vi "Create Unique SheetID.vi"(8 "error in":errorcluster, 11 "Sheets in":refnum<k24>) -> (0 "error out":errorcluster, 2 "Unique SheetID":u32, 3 "Sheets out":refnum<k24>)   [LabVIEW 2019, in "Open Xml.lvlib"]
uses:
  Open Xml.lvlib
  D:/git/Open-Xml-LabVIEW/Source/DocumentFormat.OpenXml.dll
  DocumentFormat.OpenXml.dll
  D:/git/Open-Xml-LabVIEW/Source/DocumentFormat.OpenXml.Framework.dll
  DocumentFormat.OpenXml.Framework.dll
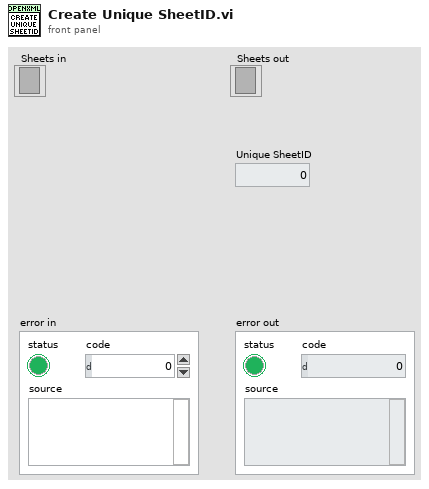
[diagram p1: front panel]
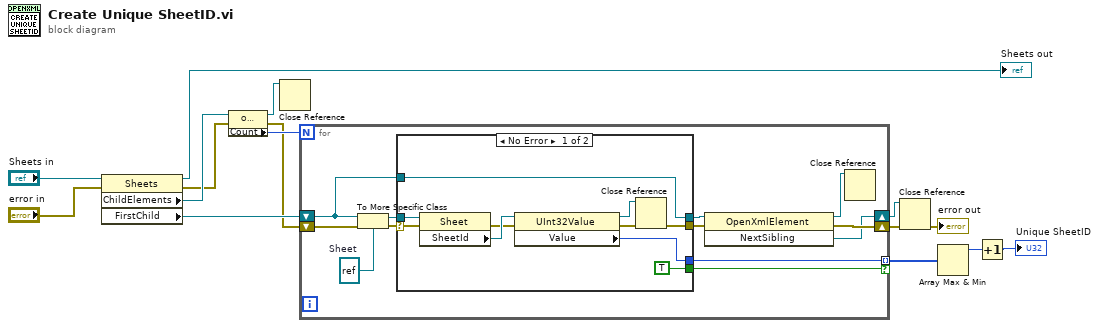
[diagram p0: block diagram]
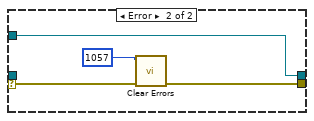
[diagram p2: hidden frame]
diagram:
  n1 = property class="Sheets"(reference="Sheets in", error in="error in") -> (reference out=→"Sheets out":refnum<k24>, error out=w9:errorcluster, "ChildElements"=w14:refnum<k24>, "FirstChild"=w11:refnum<k24>)
  n2 = property class="OpenXmlElementList"(reference=w14, error in=w9) -> (reference out=w4:refnum<k24>, error out=w10:errorcluster, "Count"=w12:i32)
  n3 = Close Reference(reference=w4) -> ()  [unwired: 1 in, 1 out]
  n4 = for {
    N: w12 -> [_]
    tunnel: [w24] -> w8 mode=indexing if=w23
    shift-right: [w20] -> w5
    shift-left: w10 -> [w19]
    shift-right: [w16] -> w1
    shift-left: w11 -> [w18]
    w27 = refnum<k24> refnum  # Sheet
    n5 = To More Specific Class(target class=w27, reference=w18, error in=w19) -> (specific class reference=w25:refnum<k24>, error out=w26:errorcluster)
    n6 = case shown="No Error" w26 {
      selector: w26 -> [w34 w41]
      tunnel: w25 -> [w37 _]
      tunnel: [w28 _] -> w24
      tunnel: [TRUE _] -> w23
      tunnel: [w30 w40] -> w22
      tunnel: [w33 w38] -> w21
      tunnel: w18 -> [w33 w38]
      frame No Error {
        n7 = property class="Sheet"(reference=w37, error in=w34) -> (error out=w32:errorcluster, "SheetId"=w36:refnum<k24>)  [unwired: 1 out]
        n8 = property class="UInt32Value"(reference=w36, error in=w32) -> (reference out=w29:refnum<k24>, error out=w31:errorcluster, "Value"=w28:u32)
        n9 = Close Reference(reference=w29, error in (no error)=w31) -> (error out=w30:errorcluster)
      }
      frame Error {
        n10 = call <vilib>:"Clear Errors.vi"("error in (no error)"=w41, "specific error code to clear (0: all)"=1057) -> ("error out"=w40:errorcluster)  [unwired: 4 in, 1 out]
      }
    }
    n11 = invoke class="OpenXmlElement" method="NextSibling"(reference=w21, error in=w22) -> (reference out=w17:refnum<k24>, error out=w20:errorcluster, "NextSibling"=w16:refnum<k24>)  [unwired: 1 in]
    n12 = Close Reference(reference=w17) -> ()  [unwired: 1 in, 1 out]
  }
  n13 = Close Reference(reference=w1, error in (no error)=w5) -> (error out=→"error out":errorcluster)
  n14 = Array Max & Min(array=w8) -> (max value=w7:u32)  [unwired: 3 out]
  n15 = Increment(x=w7) -> (x+1=→"Unique SheetID":u32)
